vi "ReadHTML.vi"(11 "url":string="http://localhost:8000") -> (0 "error out":errorcluster, 1 "path":string, 3 "Info":T1)   [LabVIEW 2019]
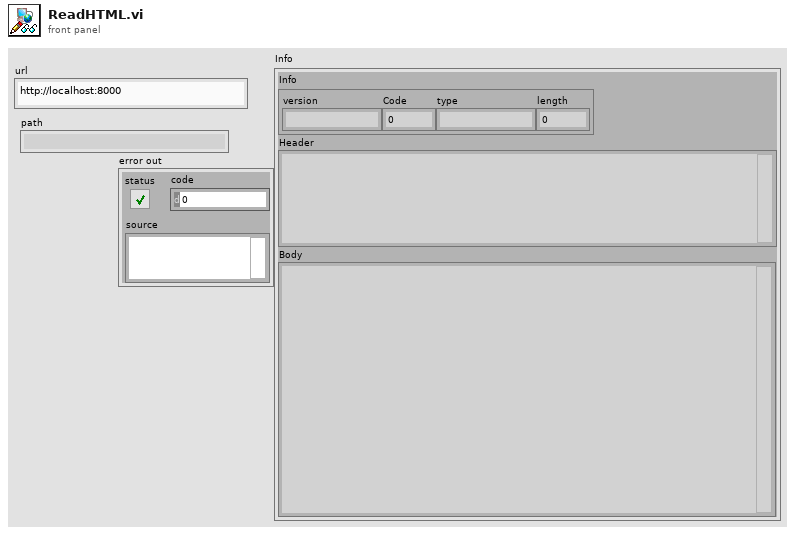
[diagram p1: front panel]
types:
  T1 = cluster{"Info":cluster{"version":string, "Code":i32, "type":string, "length":i32}, "Header":string, "Body":string}
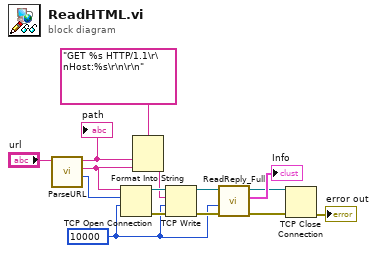
[diagram p0: block diagram]
diagram:
  w9 = 10000 ("timeout ms (60000)")
  n1 = call "ParseURL.vi"("url"="url") -> ("port"=w7:i32, "base url"=w6:string, "path"=w5:string)  [unwired: 8 in]
  "path" <- w5
  n2 = TCP Open Connection(address=w6, remote port or service name=w7, timeout ms (60000)=w9) -> (connection ID=w15:refnum<k5>, error out=w13:errorcluster)  [unwired: 2 in]
  n3 = Format Into String(format string="GET %s HTTP/1.1\r\nHost:%s\r\n\r\n", w5, w6) -> (resulting string=w14:string)  [unwired: 2 in, 1 out]
  n4 = TCP Write(connection ID=w15, data in=w14, error in (no error)=w13, 9:w9) -> (connection ID out=w11:refnum<k5>, error out=w12:errorcluster)  [unwired: 1 out]
  n5 = call "ReadReply_Full.vi"("error in (no error)"=w12, "timeout ms (60000)"=w9, "TCP in"=w11) -> ("error out"=w2:errorcluster, "Info"=→"Info":T1, "TCP out"=w3:refnum<k5>)  [unwired: 6 in]
  n6 = TCP Close Connection(connection ID=w3, error in (no error)=w2) -> (error out=→"error out":errorcluster)  [unwired: 1 in, 1 out]
